vi "pco.camera_SaveImages_Example_IMAQ.vi"() -> ()   [LabVIEW 2019]
uses:
  pco.camera/Camera.lvclass
panel:
  out "rawImage":u16[][](array[numeric])
  out "Image":T1(plugin-control)
  in  "data_format":T2(ring)=enum."Mono16"
  in  "Image Index":u32 max=9
  in  "saveImages":bool
  in  "SavePath":path
  out "Recorded Images":u32
  in  "Quit":bool
  in  "roiY1":u64=2 min=1 max=1040 step=1
  in  "roiX1":u64=2 min=1 max=1392 step=1
  in  "roiY0":u64=1 max=1039 step=1
  in  "roiX0":u64=1 max=1391 step=1
  out "Image Height":u16
  out "Image Width":u16
  in  "dwImgCount":u32=10 caption="Required Number of Images" max=4023
  out "Error":errorcluster {"code" format="%x"}
  # "This example shows how to record an image sequence and save all images to files (and an .avi) afterwards.\nIt is a good starting point for writing own applications with file saving\nBut it will not be fail save, i.e. doesnt react on errors, just handles them forward to the end\n\nUsage:\nSelect your required image count you want to record before you start the program.\nOnce started, the camera class will be initialized and images will be recorded automatically.\nWhen acquisition has finished you can read the images by index, crop them using the ROI parameters and select a file path.\nBy clicking save, the images are saved with the selected file format using the current active roi setting.\nThis also finishes the program and will force an exit of the camera class"
  # "pco.labview"
  # "Camera Setup"
  # "Recording Control"
  # "Parameters for image readout"
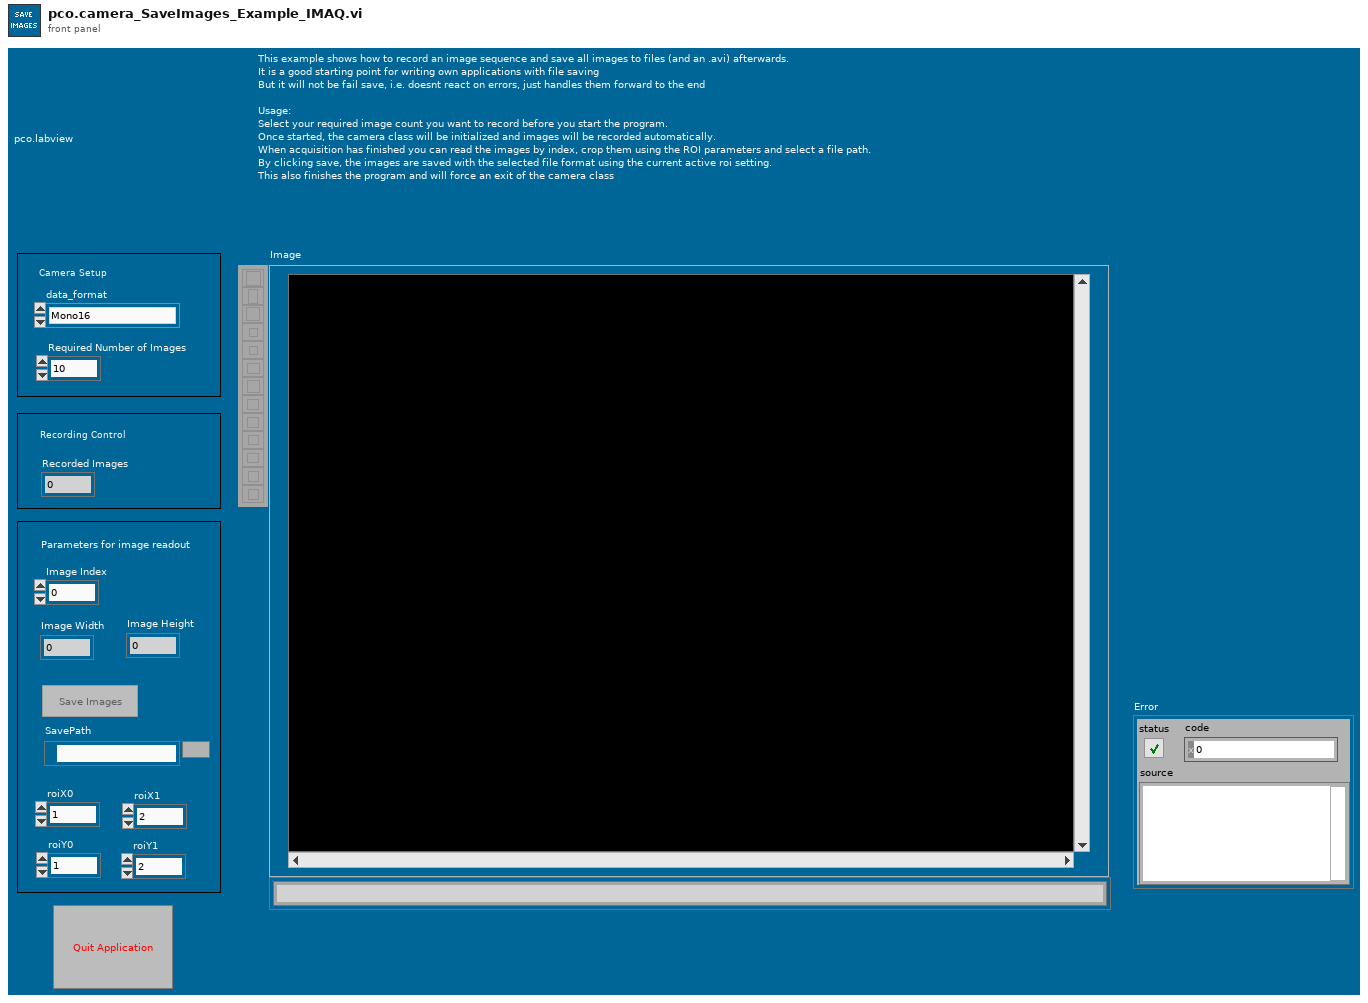
[diagram p1: front panel]
types:
  T1 = typedef "IMAQ Image.ctl" = refnum<image>
  T2 = enum16{"Undefined", "Mono8", "Mono16", "BGRA8", "RGBA8", "BGRA16", "RGBA16", "CompressedMono8"}
  T3 = enum8{"Enabled", "Disabled", "Disabled and Grayed Out"}
  T4 = enum16{"sequence", "sequence non blocking", "ring buffer", "fifo", "sequence_dpcore", "sequence_non_blocking_dpcore", "ring_buffer_dpcore", "fifo_dpcore", "tif", "multitif", "pcoraw", "b16", "dicom", "multidicom"}
  T5 = cluster{"serial":u32, "type":u16, "sub_type":u16, "interface_type":u16, "bit_resolution":u16, "min_exposure_time_s":dbl, "max_exposure_time_s":dbl, "min_exposure_step_s":dbl, "min_delay_time_s":dbl, "max_delay_time_s":dbl, "min_delay_step_s":dbl, "min_width":u64, "min_height":u64, "max_width":u64, "max_height":u64, "roi_step_horz":u64, "roi_step_vert":u64, "roi_symmetric_horz":bool, "roi_symmetric_vert":bool, "has_timestamp_mode":bool, "has_timestamp_mode_ascii_only":bool, "pixelrate_vec":u32[], "has_acquire_mode":bool, "has_ext_acquire_mode":bool, "has_metadata_mode":bool, "has_ram":bool, "binning_horz_vec":u16[], "binning_vert_vec":u16[]}
  T6 = typedef "Image Type" = u32
  T7 = typedef "Camera.lvclass/binning.ctl" = cluster{"vert":u16, "horz":u16}
  T8 = cluster{"exposure_time_s":dbl, "delay_time_s":dbl, "roi":cluster{"x0":u64, "y0":u64, "x1":u64, "y1":u64}, "timestamp_mode":u16, "pixelrate":u32, "trigger_mode":u16, "acquire_mode":u16, "metadata_mode":u16, "noisefilter_mode":u16, "binning":T7}
  T9 = cluster{"Plane 4 (alpha)":u16, "Plane 1 (Red)":u16, "Plane 2 (Green)":u16, "Plane 3 (Blue)":u16}[][]
  T10 = cluster{"dwImgCounter":u32, "lvTimestamp":timestamp, "dwMicroSeconds":u32}[]
  T11 = cluster{"Plane 4 (alpha)":u16, "Plane 1 (Red)":u16, "Plane 2 (Green)":u16, "Plane 3 (Blue)":u16}[][][]
  T12 = cluster{"dwImgCounter":u32, "lvTimestamp":timestamp, "dwMicroSeconds":u32}
  T13 = typedef "IMAQ AVI2 Refnum.ctl" = refnum<k20>
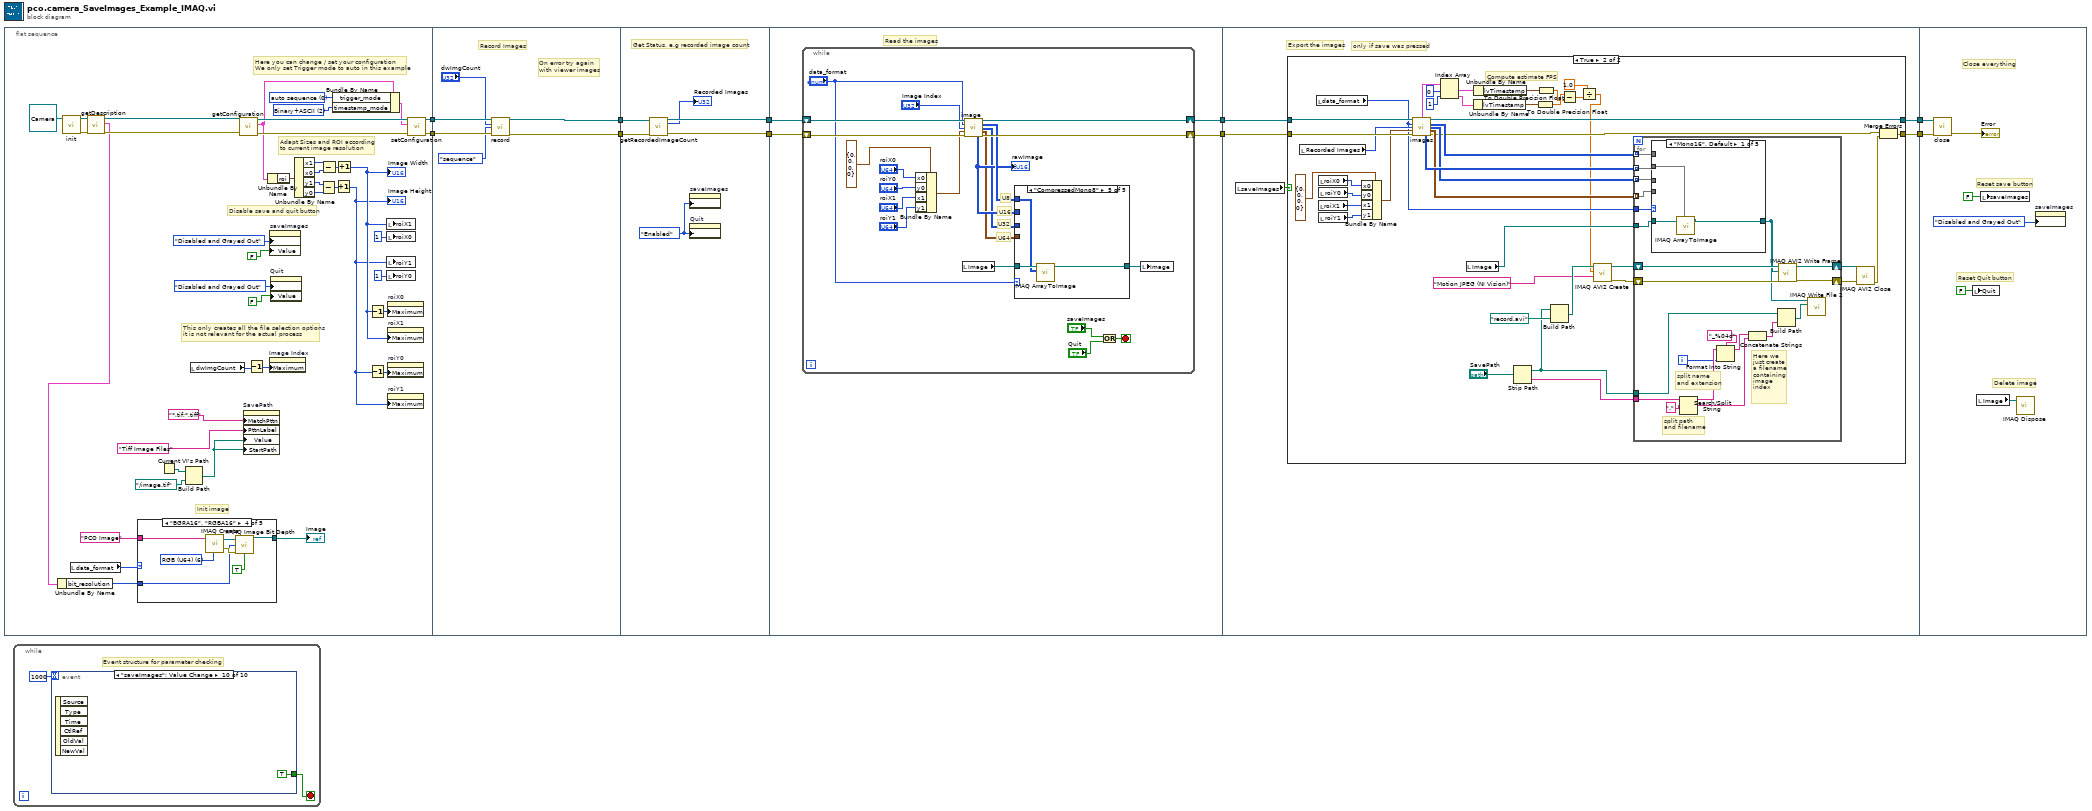
[diagram p0: block diagram]
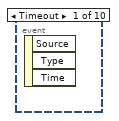
[diagram p2: hidden frame]
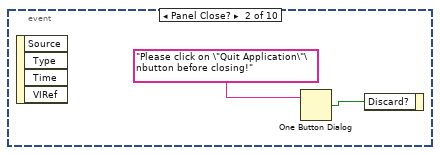
[diagram p3: hidden frame]
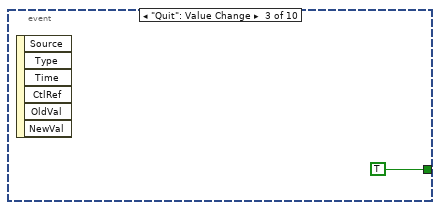
[diagram p4: hidden frame]
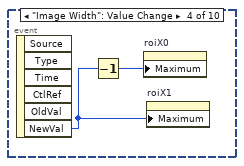
[diagram p5: hidden frame]
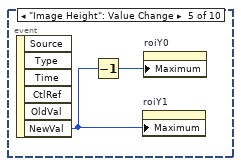
[diagram p6: hidden frame]
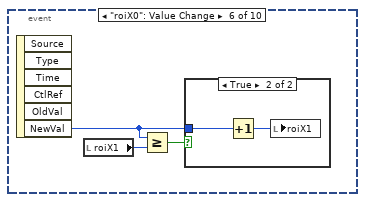
[diagram p7: hidden frame]
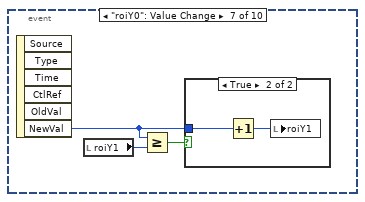
[diagram p9: hidden frame]
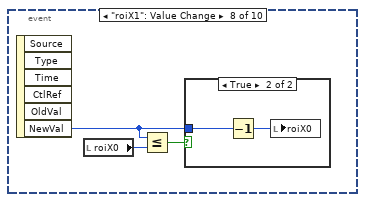
[diagram p11: hidden frame]
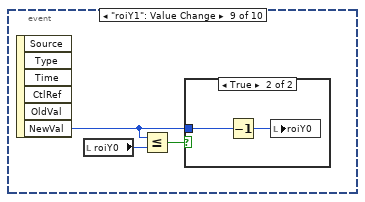
[diagram p13: hidden frame]
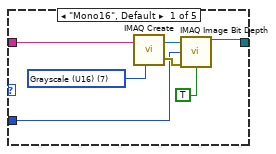
[diagram p15: hidden frame]
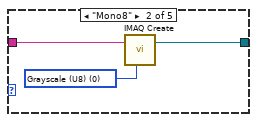
[diagram p16: hidden frame]
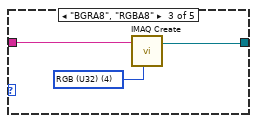
[diagram p17: hidden frame]
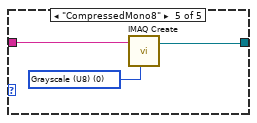
[diagram p18: hidden frame]
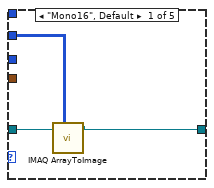
[diagram p19: hidden frame]
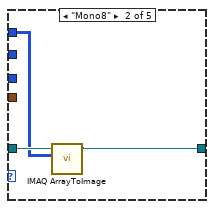
[diagram p20: hidden frame]
diagram:
  n1 = flat-sequence {
    tunnel: [w45] -> w10
    tunnel: [w44] -> w9
    tunnel: w10 -> [w81]
    tunnel: w9 -> [w80]
    tunnel: [w78] -> w8
    tunnel: [w77] -> w7
    tunnel: w8 -> [w87]
    tunnel: w7 -> [w86]
    tunnel: [w85] -> w6
    tunnel: [w84] -> w5
    tunnel: w6 -> [w90]
    tunnel: w5 -> [w91]
    tunnel: [w89] -> w4
    tunnel: [w88] -> w2
    tunnel: w4 -> [w131]
    tunnel: [w130] -> w3
    tunnel: w2 -> [w129]
    tunnel: [w128] -> w1
    tunnel: w3 -> [w218]
    tunnel: w1 -> [w217]
    frame #0 {
      w29 = u16 2 items=["OFF", "Binary", "Binary+ASCII", "ASCII"] ("TimestampMode")
      w51 = u16 0 items=["auto sequence"=0, "software trigger"=1, "external exposure start & software trigger"=2, "external exposure control"=3, "external synchronized"=4, "fast external exposure control"=5, "external CDS control"=6, "slow external exposure control"=7, "external synchronized HDSDI"=258] ("TriggerMode")
      # "Init image"
      # "This only creates all the file selection options\nit is not relevant for the actual process"
      # "Adapt Sizes and ROI according\nto current image resolution"
      # "Disable save and quit button"
      # "Here you can change / set your configuration\nWe only set Trigger mode to auto in this example"
      n2 = call-dynamic "init.vi"("Camera in"=refnum<class "Camera.lvclass"> refnum ("PCOCamera in")) -> ("Camera out"=w15:refnum<class "Camera.lvclass">, "error out"=w16:errorcluster)  [unwired: 8 in]
      n3 = local read "data_format"() -> (w19:T2)
      n4 = call-dynamic "getDescription.vi"("error in (no error)"=w16, "Camera in"=w15) -> ("error out"=w14:errorcluster, "description"=w12:T5, "Camera out"=w13:refnum<class "Camera.lvclass">)  [unwired: 7 in]
      n5 = Unbundle By Name(w12) -> ("bit_resolution"=w11:u16)
      n6 = case shown="\"BGRA16\", \"RGBA16\"" w19 {
        tunnel: "PCO Image" ("Image Name") -> [w58 w62 w64 w71 w74]
        tunnel: [w54 w60 w63 w68 w73] -> w18
        tunnel: w11 -> [w53 _ _ w66 _]
        frame "Mono16", Default {
          w59 = T6 7 items=["Grayscale (U8)", "Grayscale (I16)", "Grayscale (SGL)", "Complex (CSG)", "RGB (U32)", "HSL (U32)", "RGB (U64)", "Grayscale (U16)"] ("Image Type")
          n7 = call "IMAQ Create"("Image Name"=w58, "Image Type"=w59) -> ("New Image"=w57:T1, "error out"=w56:errorcluster)  [unwired: 3 in]
          n8 = call "IMAQ Image Bit Depth"("Image"=w57, "Bit Depth (0)"=w53, "error in (no error)"=w56, "Get/Set Bit Depth? (Set)"=TRUE) -> ("Image Out"=w54:T1)  [unwired: 9 in, 2 out]
        }
        frame "Mono8" {
          w61 = T6 0 items=["Grayscale (U8)", "Grayscale (I16)", "Grayscale (SGL)", "Complex (CSG)", "RGB (U32)", "HSL (U32)", "RGB (U64)", "Grayscale (U16)"] ("Image Type")
          n9 = call "IMAQ Create"("Image Name"=w62, "Image Type"=w61) -> ("New Image"=w60:T1)  [unwired: 3 in, 1 out]
        }
        frame "BGRA8", "RGBA8" {
          w65 = T6 4 items=["Grayscale (U8)", "Grayscale (I16)", "Grayscale (SGL)", "Complex (CSG)", "RGB (U32)", "HSL (U32)", "RGB (U64)", "Grayscale (U16)"] ("Image Type")
          n10 = call "IMAQ Create"("Image Name"=w64, "Image Type"=w65) -> ("New Image"=w63:T1)  [unwired: 3 in, 1 out]
        }
        frame "BGRA16", "RGBA16" {
          w72 = T6 6 items=["Grayscale (U8)", "Grayscale (I16)", "Grayscale (SGL)", "Complex (CSG)", "RGB (U32)", "HSL (U32)", "RGB (U64)", "Grayscale (U16)"] ("Image Type")
          n11 = call "IMAQ Create"("Image Name"=w71, "Image Type"=w72) -> ("New Image"=w69:T1, "error out"=w67:errorcluster)  [unwired: 3 in]
          n12 = call "IMAQ Image Bit Depth"("Image"=w69, "Bit Depth (0)"=w66, "error in (no error)"=w67, "Get/Set Bit Depth? (Set)"=TRUE) -> ("Image Out"=w68:T1)  [unwired: 9 in, 2 out]
        }
        frame "CompressedMono8" {
          w75 = T6 0 items=["Grayscale (U8)", "Grayscale (I16)", "Grayscale (SGL)", "Complex (CSG)", "RGB (U32)", "HSL (U32)", "RGB (U64)", "Grayscale (U16)"] ("Image Type")
          n13 = call "IMAQ Create"("Image Name"=w74, "Image Type"=w75) -> ("New Image"=w73:T1)  [unwired: 3 in, 1 out]
        }
      }
      "Image" <- w18
      n14 = Current VI's Path() -> (path=w26:path)
      n15 = Build Path(base path=w26, name or relative path=path "../image.tif" ("SavePath")) -> (appended path=w23:path)
      n16 = local read "dwImgCount"() -> (w21:u32)
      n17 = call-dynamic "getConfiguration.vi"("error in (no error)"=w14, "Camera in"=w13) -> ("error out"=w49:errorcluster, "configuration"=w39:T8, "Camera out"=w50:refnum<class "Camera.lvclass">)  [unwired: 7 in]
      n18 = property on="SavePath" class="Path"("MatchPttn"="*.tif;*.tiff" ("pattern (all files)"), "PttnLabel"="Tiff Image Files" ("pattern label"), "Value"=w23, "StartPath"=w23) -> ()  [unwired: 2 in, 2 out]
      n19 = Decrement(x=w21) -> (x-1=w22:u32)
      n20 = Unbundle By Name(w39) -> ("roi"=w38:cluster{"x0":u64, "y0":u64, "x1":u64, "y1":u64})
      n21 = property on="Image Index" class="DigNum (strict)"("Maximum"=w22) -> ()  [unwired: 2 in, 2 out]
      n22 = property on="saveImages" class="Bool (strict)"("DisabledEnum"=T3."Disabled and Grayed Out" ("Disabled"), "Value"=FALSE ("Stop")) -> ()  [unwired: 2 in, 2 out]
      n23 = property on="Quit" class="Bool (strict)"("DisabledEnum"=T3."Disabled and Grayed Out" ("Disabled"), "Value"=FALSE ("Stop")) -> ()  [unwired: 2 in, 2 out]
      n24 = Unbundle By Name(w38) -> ("x1"=w36:u64, "x0"=w37:u64, "y1"=w34:u64, "y0"=w35:u64)
      n25 = Subtract(x=w34, y=w35) -> (x-y=w32:u64)
      n26 = Subtract(x=w36, y=w37) -> (x-y=w33:u64)
      n27 = Bundle By Name(cluster=w39, "trigger_mode"=w51, "timestamp_mode"=w29) -> (w48:T8)
      n28 = Increment(x=w32) -> (x+1=w30:u64)
      "Image Height" <- w30
      n29 = Increment(x=w33) -> (x+1=w31:u64)
      "Image Width" <- w31
      n30 = Decrement(x=w31) -> (x-1=w41:u64)
      n31 = Decrement(x=w30) -> (x-1=w40:u64)
      n32 = local write "roiX1"(w31) -> ()
      n33 = local write "roiX0"(u16 1 ("roiY0")) -> ()
      n34 = local write "roiY1"(w30) -> ()
      n35 = local write "roiY0"(u16 1 ("roiY0")) -> ()
      n36 = property on="roiX0" class="DigNum (strict)"("Maximum"=w41) -> ()  [unwired: 2 in, 2 out]
      n37 = property on="roiX1" class="DigNum (strict)"("Maximum"=w31) -> ()  [unwired: 2 in, 2 out]
      n38 = property on="roiY0" class="DigNum (strict)"("Maximum"=w40) -> ()  [unwired: 2 in, 2 out]
      n39 = property on="roiY1" class="DigNum (strict)"("Maximum"=w30) -> ()  [unwired: 2 in, 2 out]
      n40 = call-dynamic "setConfiguration.vi"("error in (no error)"=w49, "configuration"=w48, "Camera in"=w50) -> ("error out"=w44:errorcluster, "Camera out"=w45:refnum<class "Camera.lvclass">)  [unwired: 7 in]
    }
    frame #1 {
      # "On error try again \nwith viewer images"
      # "Record Images"
      n41 = call-dynamic "record.vi"("Camera in"=w81, "num_images"="dwImgCount", "record_mode"=T4."sequence", "error in (no error)"=w80) -> ("Camera out"=w78:refnum<class "Camera.lvclass">, "error out"=w77:errorcluster)  [unwired: 10 in]
    }
    frame #2 {
      w82 = T3."Enabled" ("Disabled")
      # "Get Status, e.g recorded image count"
      n42 = call-dynamic "getRecordedImageCount.vi"("Camera in"=w87, "error in (no error)"=w86) -> ("Camera out"=w85:refnum<class "Camera.lvclass">, "recorded_image_count"=→"Recorded Images":u32, "error out"=w84:errorcluster)  [unwired: 11 in]
      n43 = property on="saveImages" class="Bool (strict)"("DisabledEnum"=w82) -> ()  [unwired: 2 in, 2 out]
      n44 = property on="Quit" class="Bool (strict)"("DisabledEnum"=w82) -> ()  [unwired: 2 in, 2 out]
    }
    frame #3 {
      # "Read the images"
      n45 = while {
        shift-right: [w110] -> w89
        shift-left: w90 -> [w112]
        shift-right: [w105] -> w88
        shift-left: w91 -> [w111]
        stop <- w103 stop-if-true
        # "U64"
        # "U32"
        # "U16"
        # "U8"
        n46 = Bundle By Name(cluster=cluster{"x0":u64, "y0":u64, "x1":u64, "y1":u64} {"x0"=0, "y0"=0, "x1"=0, "y1"=0} ("roi"), "x0"="roiX0", "y0"="roiY0", "x1"="roiX1", "y1"="roiY1") -> (w101:cluster{"x0":u64, "y0":u64, "x1":u64, "y1":u64})
        n47 = local read "Image"() -> (w94:T1)
        n48 = call-dynamic "image.vi"("Camera in"=w112, "data_format"="data_format", "image_index"="Image Index", "roi"=w101, "error in (no error)"=w111) -> ("Camera out"=w110:refnum<class "Camera.lvclass">, "image (U8)"=w98:u8[][], "image (U32)"=w96:u32[][], "image (U64)"=w95:T9, "raw_image (U16)"=w97:u16[][], "error out"=w105:errorcluster)  [unwired: 3 in, 2 out]
        "rawImage" <- w97
        n49 = case shown="\"CompressedMono8\"" "data_format" {
          tunnel: w94 -> [w115 w118 w121 w124 w127]
          tunnel: [w113 w116 w120 w122 w126] -> w93
          tunnel: w95 -> [_ _ _ w123 _]
          tunnel: w96 -> [_ _ w119 _ _]
          tunnel: w98 -> [_ w117 _ _ w125]
          tunnel: w97 -> [w114 _ _ _ _]
          frame "Mono16", Default {
            n50 = call "IMAQ ArrayToImage"("Image Pixels (U16)"=w114, "Image"=w115) -> ("Image Out"=w113:T1)  [unwired: 8 in, 1 out]
          }
          frame "Mono8" {
            n51 = call "IMAQ ArrayToImage"("Image Pixels (U8)"=w117, "Image"=w118) -> ("Image Out"=w116:T1)  [unwired: 8 in, 1 out]
          }
          frame "BGRA8", "RGBA8" {
            n52 = call "IMAQ ArrayToColorImage"("Image Pixels (U32)"=w119, "Image"=w121) -> ("Image Out"=w120:T1)  [unwired: 3 in, 1 out]
          }
          frame "BGRA16", "RGBA16" {
            n53 = call "IMAQ ArrayToColorImage"("Image"=w124, "Image Pixels (U64)"=w123) -> ("Image Out"=w122:T1)  [unwired: 3 in, 1 out]
          }
          frame "CompressedMono8" {
            n54 = call "IMAQ ArrayToImage"("Image Pixels (U8)"=w125, "Image"=w127) -> ("Image Out"=w126:T1)  [unwired: 8 in, 1 out]
          }
        }
        n55 = Or(x="saveImages", y="Quit") -> (x .or. y?=w103:bool)
        n56 = local write "Image"(w93) -> ()
      }
    }
    frame #4 {
      # "only if save was pressed"
      # "Export the images"
      n57 = local read "saveImages"() -> (w132:bool)
      n58 = case shown="True" w132 {
        tunnel: w131 -> [w134 w174]
        tunnel: [w134 w162] -> w130
        tunnel: w129 -> [w133 w175]
        tunnel: [w133 w155] -> w128
        frame False {
        }
        frame True {
          # "Compute estimate FPS"
          n59 = local read "Recorded Images"() -> (w167:u32)
          n60 = local read "data_format"() -> (w153:T2)
          n61 = local read "roiX0"() -> (w172:u64)
          n62 = local read "roiX1"() -> (w170:u64)
          n63 = local read "roiY0"() -> (w171:u64)
          n64 = local read "roiY1"() -> (w169:u64)
          n65 = Bundle By Name(cluster=cluster{"x0":u64, "y0":u64, "x1":u64, "y1":u64} {"x0"=0, "y0"=0, "x1"=0, "y1"=0} ("roi"), "x0"=w172, "y0"=w171, "x1"=w170, "y1"=w169) -> (w168:cluster{"x0":u64, "y0":u64, "x1":u64, "y1":u64})
          n66 = call-dynamic "images.vi"("Camera in"=w174, "data_format"=w153, "image_count"=w167, "roi"=w168, "error in (no error)"=w175) -> ("timestamp_list"=w147:T10, "Camera out"=w162:refnum<class "Camera.lvclass">, "image_list (U8)"=w166:u8[][][], "image_list (U32)"=w164:u32[][][], "image_list (U64)"=w163:T11, "raw_image_list (U16)"=w165:u16[][][], "error out"=w157:errorcluster)  [unwired: 3 in, 1 out]
          n67 = Index Array(array=w147, index #1=0 ("index"), index #2=1 ("index")) -> (element #1=w144:T12, element #2=w143:T12)
          n68 = local read "Image"() -> (w154:T1)
          n69 = Unbundle By Name(w143) -> ("lvTimestamp"=w141:timestamp)
          n70 = Unbundle By Name(w144) -> ("lvTimestamp"=w142:timestamp)
          n71 = Strip Path(path="SavePath") -> (stripped path=w148:path, name=w151:string)
          n72 = To Double Precision Float(number=w141) -> (double precision float=w140:dbl)
          n73 = To Double Precision Float(number=w142) -> (double precision float=w139:dbl)
          n74 = Build Path(base path=w148, name or relative path=path "record.avi") -> (appended path=w149:path)
          n75 = Subtract(x=w140, y=w139) -> (x-y=w138:dbl)
          n76 = Divide(x=1.0, y=w138) -> (x/y=w136:dbl)
          n77 = call "IMAQ AVI2 Create"("Codec"="Motion JPEG (NI Vision)", "Frames Per Second"=w136, "AVI Path"=w149) -> ("error out"=w161:errorcluster, "AVI Refnum"=w160:T13)  [unwired: 7 in]
          n78 = for {
            tunnel: w166 -> [w196] mode=indexing
            tunnel: w165 -> [w195] mode=indexing
            tunnel: w164 -> [w194] mode=indexing
            tunnel: w163 -> [w193] mode=indexing
            shift-right: [w189] -> w158
            shift-left: w160 -> [w192]
            shift-right: [w190] -> w159
            shift-left: w161 -> [w191]
            tunnel: w154 -> [w179]
            tunnel: w153 -> [w178]
            tunnel: w151 -> [w177]
            tunnel: w148 -> [w176]
            i -> [w181]
            # "Here we \njust create\na filename\ncontaining\nimage \nindex"
            # "split path \nand filename"
            # "split name \nand extension"
            n79 = case shown="\"Mono16\", Default" w178 {
              tunnel: w179 -> [w199 w202 w205 w208 w211]
              tunnel: [w197 w200 w204 w206 w210] -> w188
              tunnel: w193 -> [_ _ _ w207 _]
              tunnel: w194 -> [_ _ w203 _ _]
              tunnel: w196 -> [_ w201 _ _ w209]
              tunnel: w195 -> [w198 _ _ _ _]
              frame "Mono16", Default {
                n80 = call "IMAQ ArrayToImage"("Image Pixels (U16)"=w198, "Image"=w199) -> ("Image Out"=w197:T1)  [unwired: 8 in, 1 out]
              }
              frame "Mono8" {
                n81 = call "IMAQ ArrayToImage"("Image Pixels (U8)"=w201, "Image"=w202) -> ("Image Out"=w200:T1)  [unwired: 8 in, 1 out]
              }
              frame "BGRA8", "RGBA8" {
                n82 = call "IMAQ ArrayToColorImage"("Image Pixels (U32)"=w203, "Image"=w205) -> ("Image Out"=w204:T1)  [unwired: 3 in, 1 out]
              }
              frame "BGRA16", "RGBA16" {
                n83 = call "IMAQ ArrayToColorImage"("Image"=w208, "Image Pixels (U64)"=w207) -> ("Image Out"=w206:T1)  [unwired: 3 in, 1 out]
              }
              frame "CompressedMono8" {
                n84 = call "IMAQ ArrayToImage"("Image Pixels (U8)"=w209, "Image"=w211) -> ("Image Out"=w210:T1)  [unwired: 8 in, 1 out]
              }
            }
            n85 = Search/Split String(string=w177, search string/char (-)=".") -> (substring before match=w185:string, match + rest of string=w186:string)  [unwired: 1 in, 1 out]
            n86 = Format Into String(format string="_%04d", initial string=w185, w181) -> (resulting string=w187:string)  [unwired: 1 in, 1 out]
            n87 = Concatenate Strings(w187, w186) -> (w182:string)
            n88 = Build Path(base path=w176, name or relative path=w182) -> (appended path=w180:path)
            n89 = call "IMAQ AVI2 Write Frame"("error in (no error)"=w191, "Image"=w188, "AVI Refnum"=w192) -> ("error out"=w190:errorcluster, "AVI Refnum (duplicate)"=w189:T13)  [unwired: 6 in, 1 out]
            n90 = call-poly "IMAQ Write File 2"("File Path"=w180, "Image"=w188) -> ()  [unwired: 8 in, 2 out]
          }
          n91 = call "IMAQ AVI2 Close"("error in (no error)"=w159, "AVI Refnum"=w158) -> ("error out"=w156:errorcluster)  [unwired: 9 in]
          n92 = Merge Errors(w157, w156) -> (w155:errorcluster)
        }
      }
    }
    frame #5 {
      # "Delete image"
      # "Reset Quit button"
      # "Close everything"
      # "Reset save button"
      n93 = call-dynamic "close.vi"("error in (no error)"=w217, "Camera in"=w218) -> ("error out"=→"Error":errorcluster)  [unwired: 9 in]
      n94 = local write "Quit"(FALSE ("Stop")) -> ()
      n95 = local read "Image"() -> (w212:T1)
      n96 = local write "saveImages"(FALSE ("Stop")) -> ()
      n97 = call "IMAQ Dispose"("Image"=w212) -> ()  [unwired: 5 in, 1 out]
      n98 = property on="saveImages" class="Bool (strict)"("DisabledEnum"=T3."Disabled and Grayed Out" ("Disabled")) -> ()  [unwired: 2 in, 2 out]
    }
  }
  n99 = while {
    stop <- w219 stop-if-true
    # "Event structure for parameter checking"
    n100 = event shown="[9] \"saveImages\": Value Change" {
      selector: _ -> [_ _ _ _ _ _ _ _ _ _]
      dyn-events: _ -> [_ _ _ _ _ _ _ _ _ _]
      timeout: 1000 -> [_ _ _ _ _ _ _ _ _ _]
      tunnel: [_ _ TRUE _ _ _ _ _ _ TRUE] -> w219
      event Timeout {
        n101 = event-data() -> ()  [unwired: 1 in, 3 out]
      }
      event Panel Close? {
        n102 = event-data() -> ()  [unwired: 1 in, 4 out]
        n103 = One Button Dialog(message="Please click on \"Quit Application\"\nbutton before closing!") -> (true=w221:bool)  [unwired: 1 in]
        n104 = event-data("Discard?"=w221) -> ()  [unwired: 1 in, 1 out]
      }
      event "Quit": Value Change {
        n105 = event-data() -> ()  [unwired: 1 in, 6 out]
      }
      event "Image Width": Value Change {
        n106 = event-data() -> ("NewVal"=w224:u16)  [unwired: 1 in, 5 out]
        n107 = Decrement(x=w224) -> (x-1=w225:u16)
        n108 = property on="roiX0" class="DigNum (strict)"("Maximum"=w225) -> ()  [unwired: 2 in, 2 out]
        n109 = property on="roiX1" class="DigNum (strict)"("Maximum"=w224) -> ()  [unwired: 2 in, 2 out]
      }
      event "Image Height": Value Change {
        n110 = event-data() -> ("NewVal"=w226:u16)  [unwired: 1 in, 5 out]
        n111 = Decrement(x=w226) -> (x-1=w227:u16)
        n112 = property on="roiY1" class="DigNum (strict)"("Maximum"=w226) -> ()  [unwired: 2 in, 2 out]
        n113 = property on="roiY0" class="DigNum (strict)"("Maximum"=w227) -> ()  [unwired: 2 in, 2 out]
      }
      event "roiX0": Value Change {
        n114 = event-data() -> ("NewVal"=w228:u64)  [unwired: 1 in, 5 out]
        n115 = local read "roiX1"() -> (w230:u64)
        n116 = Greater Or Equal?(x=w228, y=w230) -> (x >= y?=w229:bool)
        n117 = case shown="True" w229 {
          tunnel: w228 -> [_ w232]
          frame False {
          }
          frame True {
            n118 = Increment(x=w232) -> (x+1=w231:u64)
            n119 = local write "roiX1"(w231) -> ()
          }
        }
      }
      event "roiY0": Value Change {
        n120 = event-data() -> ("NewVal"=w233:u64)  [unwired: 1 in, 5 out]
        n121 = local read "roiY1"() -> (w235:u64)
        n122 = Greater Or Equal?(x=w233, y=w235) -> (x >= y?=w234:bool)
        n123 = case shown="True" w234 {
          tunnel: w233 -> [_ w237]
          frame False {
          }
          frame True {
            n124 = Increment(x=w237) -> (x+1=w236:u64)
            n125 = local write "roiY1"(w236) -> ()
          }
        }
      }
      event "roiX1": Value Change {
        n126 = event-data() -> ("NewVal"=w238:u64)  [unwired: 1 in, 5 out]
        n127 = local read "roiX0"() -> (w240:u64)
        n128 = Less Or Equal?(x=w238, y=w240) -> (x <= y?=w239:bool)
        n129 = case shown="True" w239 {
          tunnel: w238 -> [_ w242]
          frame False {
          }
          frame True {
            n130 = Decrement(x=w242) -> (x-1=w241:u64)
            n131 = local write "roiX0"(w241) -> ()
          }
        }
      }
      event "roiY1": Value Change {
        n132 = event-data() -> ("NewVal"=w243:u64)  [unwired: 1 in, 5 out]
        n133 = local read "roiY0"() -> (w245:u64)
        n134 = Less Or Equal?(x=w243, y=w245) -> (x <= y?=w244:bool)
        n135 = case shown="True" w244 {
          tunnel: w243 -> [_ w247]
          frame False {
          }
          frame True {
            n136 = Decrement(x=w247) -> (x-1=w246:u64)
            n137 = local write "roiY0"(w246) -> ()
          }
        }
      }
      event "saveImages": Value Change {
        n138 = event-data() -> ()  [unwired: 1 in, 6 out]
      }
    }
  }
